vi "Calibration_Open_One_Freq.vi"(8 "error in":errorcluster, 10 "Stop Test":bool, 11 "Calibration Test":bool) -> (0 "error out":errorcluster, 5 "Calibration Open Successful":bool)   [LabVIEW 2020]
uses:
  <vilib>/Utility/error.llb/DialogType.ctl
panel:
  out "message":string=" INSTRUCTIONS:\r\rNormal Use:  When using subVIs that incorporate the error in/error out (or error I/O) structure, place this handler where you want to inform the user of an error, typically at the end of the I/O data path, as the last action of the program.  If the error in error? is ERROR, the handler creates a message describing the error and its source.  If the type of dialog = 1 (default), the message is displayed to the user, who can only acknowedge it.  If the type = 2, the user can acknowledge the message or abort execution; aborting a program with active I/O is not recommended.  If the type = 0, no message is displayed; this is used to process the error programmatically, and the error out cluster elements are wired to individual terminals for that reason.  \r\rOther Use:\n\r\nlocal testing.  To test the error code of a subVI or function that does not have the error I/O structure, you can wire its error code and a source string to the local error code and error source inputs.  If error in error? indicates no error and error code is not equal to 0, the local code and source are substituted for the error in values, and error? is set TRUE (ERROR)."
  out "serial poll byte":i16
  in  "Cal_Delay_Step":u16
  out "Test Count":i32
  out "Failed Test Count":i32
  in  "Test Failed":bool
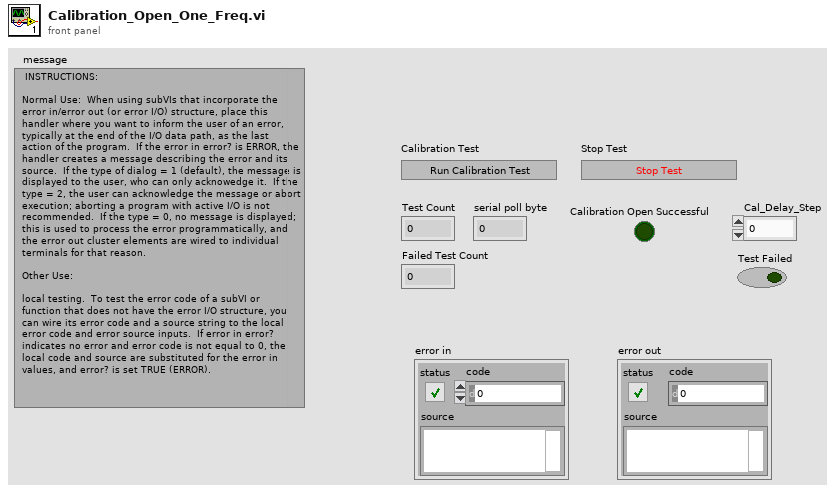
[diagram p1: front panel]
types:
  T1 = typedef "DialogType.ctl" = u16
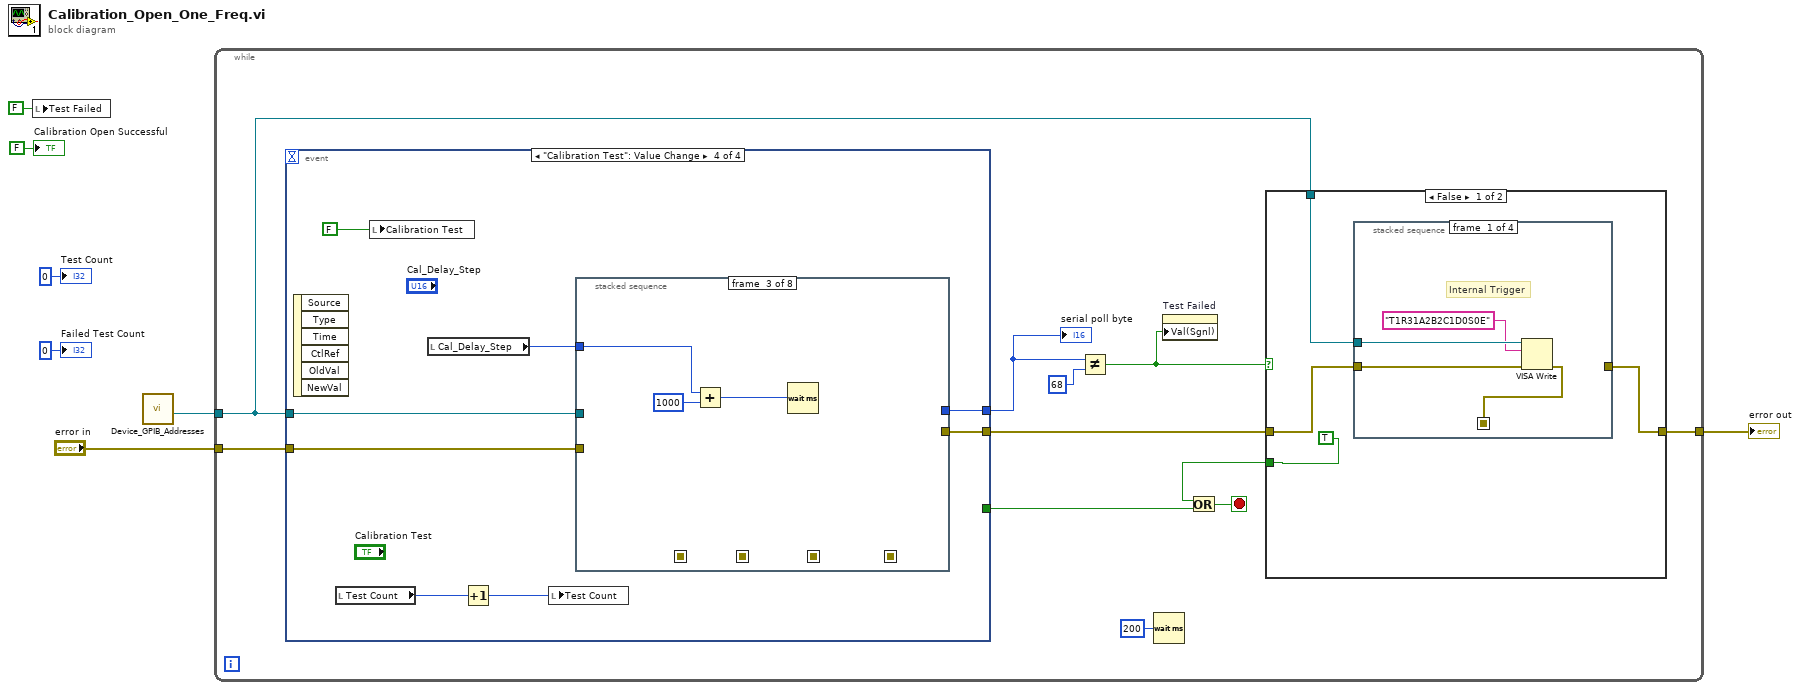
[diagram p0: block diagram]
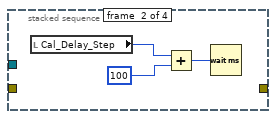
[diagram p2: hidden frame]
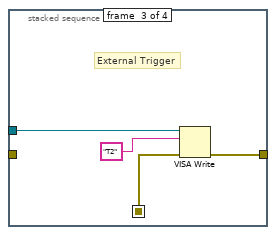
[diagram p3: hidden frame]
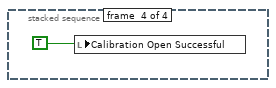
[diagram p4: hidden frame]
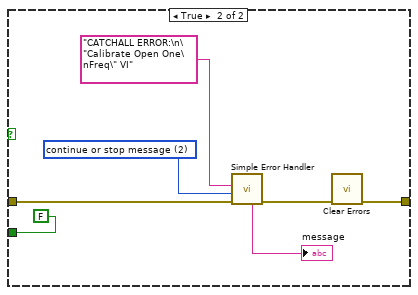
[diagram p5: hidden frame]
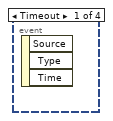
[diagram p6: hidden frame]
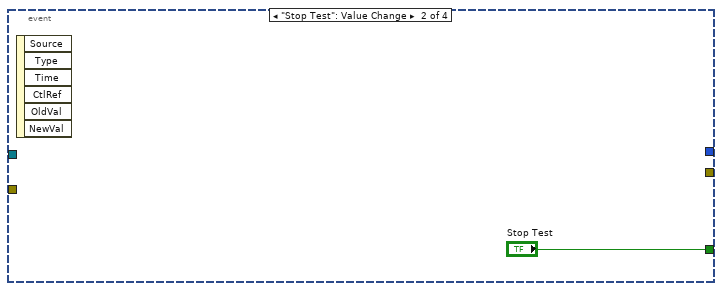
[diagram p7: hidden frame]
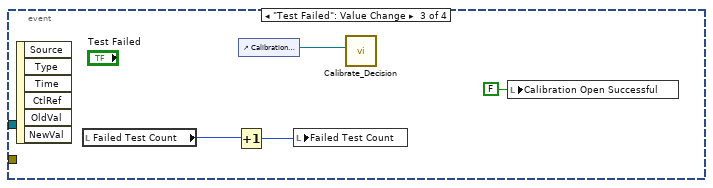
[diagram p8: hidden frame]
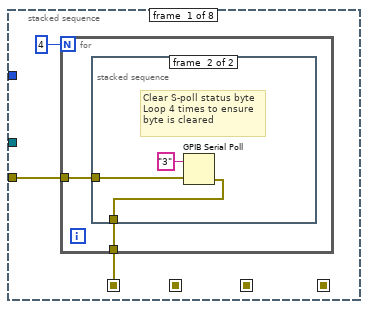
[diagram p9: hidden frame]
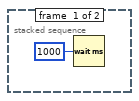
[diagram p10: hidden frame]
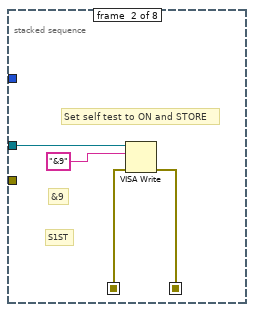
[diagram p11: hidden frame]
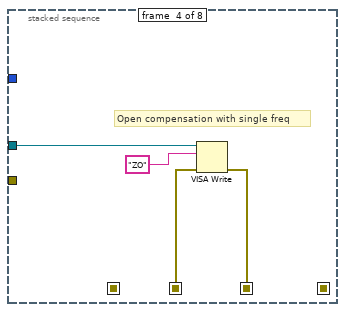
[diagram p12: hidden frame]
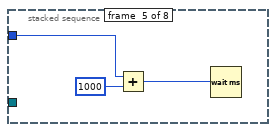
[diagram p13: hidden frame]
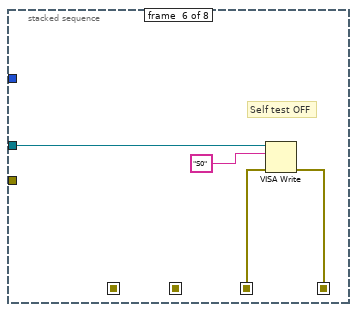
[diagram p14: hidden frame]
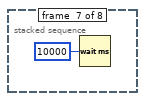
[diagram p15: hidden frame]
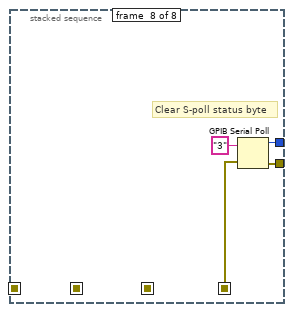
[diagram p16: hidden frame]
diagram:
  n1 = local write "Test Failed"(FALSE ("Test Failed")) -> ()
  n2 = call "Device_GPIB_Addresses.vi"() -> ("HP 4275A Address"=w5:refnum<visa-resource-name>)  [unwired: 9 in, 2 out]
  n3 = while {
    tunnel: w5 -> [w17]
    tunnel: "error in" -> [w18]
    tunnel: [w15] -> w1
    stop <- w14 stop-if-true
    n4 = event shown="[3] \"Calibration Test\": Value Change" {
      selector: _ -> [_ _ _ _]
      dyn-events: _ -> [_ _ _ _]
      timeout: _ -> [_ _ _ _]
      tunnel: [_ "Stop Test" _ _] -> w12
      tunnel: w17 -> [_ _ _ w50]
      tunnel: [_ _ _ w49] -> w16
      tunnel: w18 -> [_ _ _ w48]
      tunnel: [_ _ _ w47] -> w9
      event Timeout {
        n5 = event-data() -> ()  [unwired: 1 in, 3 out]
      }
      event "Stop Test": Value Change {
        n6 = event-data() -> ()  [unwired: 1 in, 6 out]
      }
      event "Test Failed": Value Change {
        n7 = event-data() -> ()  [unwired: 1 in, 6 out]
        n8 = local read "Failed Test Count"() -> (w44:i32)
        n9 = Increment(x=w44) -> (x+1=w45:i32)
        n10 = control-ref of="Calibration Test"() -> (w46:refnum<vi>)
        n11 = local write "Failed Test Count"(w45) -> ()
        n12 = call "Calibrate_Decision.vi"("reference"=w46) -> ()  [unwired: 11 in]
        n13 = local write "Calibration Open Successful"(FALSE ("Calibration Open Successful")) -> ()
      }
      event "Calibration Test": Value Change {
        n14 = event-data() -> ()  [unwired: 1 in, 6 out]
        n15 = local read "Test Count"() -> (w53:i32)
        n16 = local write "Calibration Test"(FALSE ("Calibration Test")) -> ()
        n17 = local read "Cal_Delay_Step"() -> (w51:u16)
        n18 = Increment(x=w53) -> (x+1=w52:i32)
        n19 = local write "Test Count"(w52) -> ()
        n20 = stacked-sequence {
          seq-local: [w55 _ _ _ _ _ _ _] -> [_ w65 _ _ _ _ _ _]
          seq-local: [_ w64 _ _ _ _ _ _] -> [_ _ _ w72 _ _ _ _]
          seq-local: [_ _ _ w71 _ _ _ _] -> [_ _ _ _ _ w79 _ _]
          seq-local: [_ _ _ _ _ w78 _ _] -> [_ _ _ _ _ _ _ w86]
          tunnel: w48 -> [w56 _ _ _ _ _ _ _]
          tunnel: w51 -> [_ _ w70 _ w75 _ _ _]
          tunnel: [_ _ _ _ _ _ _ w85] -> w49
          tunnel: [_ _ _ _ _ _ _ w84] -> w47
          tunnel: w50 -> [_ w67 _ w74 _ w80 _ _]
          frame #0 {
            n21 = for {
              N: 4 -> [_]
              tunnel: w56 -> [w59]
              tunnel: [w58] -> w55
              n22 = stacked-sequence {
                tunnel: w59 -> [_ w63]
                tunnel: [_ w62] -> w58
                frame #0 {
                  n23 = Wait (ms)(milliseconds to wait=u32 1000) -> ()  [unwired: 1 out]
                }
                frame #1 {
                  # "Clear S-poll status byte\nLoop 4 times to ensure\nbyte is cleared"
                  n24 = GPIB Serial Poll(0:"3" ("address string"), 1:w63) -> (4:w62:errorcluster)  [unwired: 2 out]
                }
              }
            }
          }
          frame #1 {
            # "S1ST"
            # "&9"
            # "Set self test to ON and STORE"
            n25 = VISA Write(VISA resource name=w67, write buffer="&9" ("data"), error in (no error)=w65) -> (error out=w64:errorcluster)  [unwired: 2 out]
          }
          frame #2 {
            n26 = Add(x=w70, y=u16 1000) -> (x+y=w68:u16)
            n27 = Wait (ms)(milliseconds to wait=w68) -> ()  [unwired: 1 out]
          }
          frame #3 {
            # "Open compensation with single freq"
            n28 = VISA Write(VISA resource name=w74, write buffer="ZO" ("data"), error in (no error)=w72) -> (error out=w71:errorcluster)  [unwired: 2 out]
          }
          frame #4 {
            n29 = Add(x=w75, y=u16 1000) -> (x+y=w76:u16)
            n30 = Wait (ms)(milliseconds to wait=w76) -> ()  [unwired: 1 out]
          }
          frame #5 {
            # "Self test OFF"
            n31 = VISA Write(VISA resource name=w80, write buffer="S0" ("data"), error in (no error)=w79) -> (error out=w78:errorcluster)  [unwired: 2 out]
          }
          frame #6 {
            n32 = Wait (ms)(milliseconds to wait=u32 10000) -> ()  [unwired: 1 out]
          }
          frame #7 {
            # "Clear S-poll status byte"
            n33 = GPIB Serial Poll(0:"3" ("address string"), 1:w86) -> (2:w84:i16, 4:w85:errorcluster)  [unwired: 1 out]
          }
        }
      }
    }
    "serial poll byte" <- w9
    n34 = Not Equal?(x=w9, y=i16 68) -> (x != y?=w11:bool)
    n35 = Wait (ms)(milliseconds to wait=u32 200) -> ()  [unwired: 1 out]
    n36 = property on="Test Failed" class="Bool (strict)"("Val(Sgnl)"=w11) -> ()  [unwired: 2 in, 2 out]
    n37 = case shown="False" w11 {
      tunnel: w17 -> [w22 _]
      tunnel: w16 -> [w21 w41]
      tunnel: [w20 w38] -> w15
      tunnel: [TRUE FALSE] -> w13
      frame False {
        n38 = stacked-sequence {
          seq-local: [w24 _ _ _] -> [_ _ w33 _]
          tunnel: w21 -> [w23 _ _ _]
          tunnel: [_ _ w31 _] -> w20
          tunnel: w22 -> [w26 _ w32 _]
          frame #0 {
            # "Internal Trigger"
            n39 = VISA Write(VISA resource name=w26, write buffer="T1R31A2B2C1D0S0E" ("Keystate"), error in (no error)=w23) -> (error out=w24:errorcluster)  [unwired: 2 out]
          }
          frame #1 {
            n40 = local read "Cal_Delay_Step"() -> (w27:u16)
            n41 = Add(x=w27, y=u16 100) -> (x+y=w28:u16)
            n42 = Wait (ms)(milliseconds to wait=w28) -> ()  [unwired: 1 out]
          }
          frame #2 {
            # "External Trigger"
            n43 = VISA Write(VISA resource name=w32, write buffer="T2" ("data"), error in (no error)=w33) -> (error out=w31:errorcluster)  [unwired: 2 out]
          }
          frame #3 {
            n44 = local write "Calibration Open Successful"(TRUE ("Open Calibration Successful")) -> ()
          }
        }
      }
      frame True {
        w37 = T1 2 items=["no dialog", "OK message", "continue or stop message", "OK message + warnings", "continue/stop + warnings"] ("type of dialog (OK msg:1)")
        n45 = call <vilib>:"Simple Error Handler.vi"("error source (\" \")"="CATCHALL ERROR:\n\"Calibrate Open One\nFreq\" VI" ("error source (\" \")"), "type of dialog (OK msg:1)"=w37, "error in (no error)"=w41) -> ("error out"=w39:errorcluster, "message"=→"message":string)  [unwired: 2 in, 3 out]
        n46 = call <vilib>:"Clear Errors.vi"("error in (no error)"=w39) -> ("error out"=w38:errorcluster)  [unwired: 5 in, 1 out]
      }
    }
    n47 = Or(x=w13, y=w12) -> (x .or. y?=w14:bool)
  }
  "error out" <- w1
  "Failed Test Count" <- 0 ("Failed Test Count")
  "Test Count" <- 0 ("Numeric")
  "Calibration Open Successful" <- FALSE ("Open Calibration Successful")
